vi "SetUpHelper.vi"(8 "ErrorIn":errorcluster, 11 "Reference":T1) -> (0 "ErrorOut":errorcluster, 3 "OutConnection":T1)   [LabVIEW 2019]
uses:
  C:/Users/user/Desktop/lvlib/assemblies/x86/LibraryForLabVIEW.dll
  assemblies/x86/LibraryForLabVIEW.dll
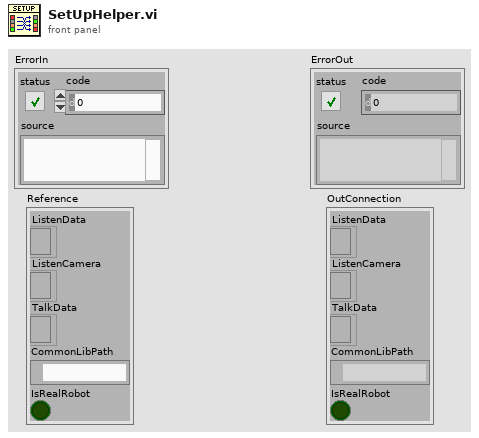
[diagram p1: front panel]
types:
  T1 = cluster{"ListenData":refnum<k24>, "ListenCamera":refnum<k24>, "TalkData":refnum<k24>, "CommonLibPath":path, "IsRealRobot":bool}
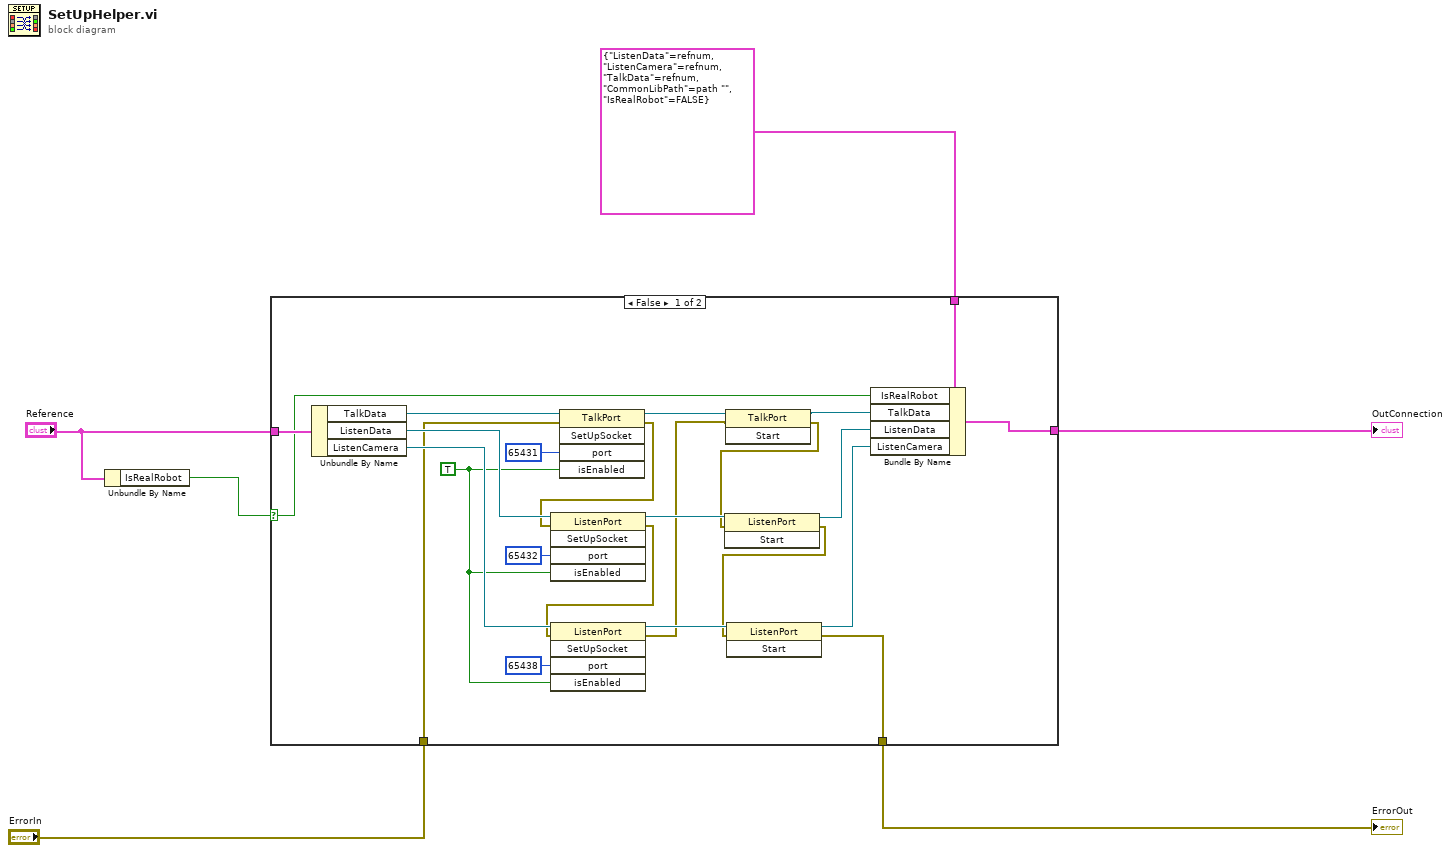
[diagram p0: block diagram]
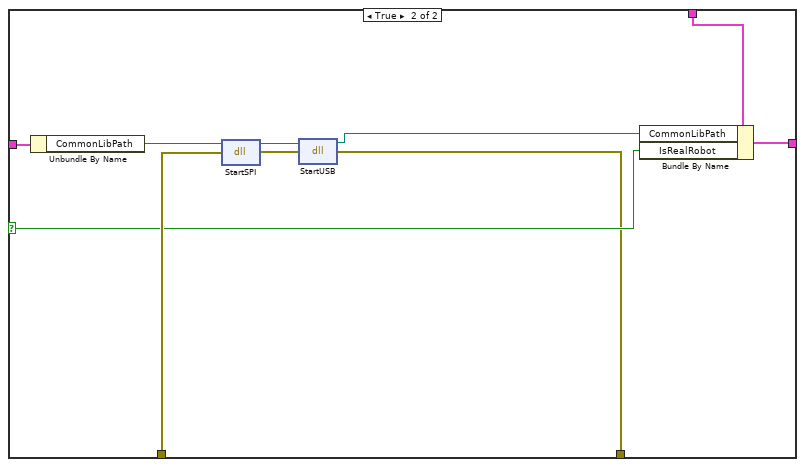
[diagram p2: hidden frame]
diagram:
  n1 = Unbundle By Name("Reference") -> ("IsRealRobot"=w1:bool)
  n2 = case shown="False" w1 {
    selector: w1 -> [w7 w35]
    tunnel: "ErrorIn" -> [w18 w38]
    tunnel: [w11 w31] -> w5
    tunnel: "Reference" -> [w10 w40]
    tunnel: T1 {"ListenData"=refnum, "ListenCamera"=refnum, "TalkData"=refnum, "CommonLibPath"=path "", "IsRealRobot"=FALSE} -> [w9 w37]
    tunnel: [w8 w36] -> w3
    frame False {
      w16 = TRUE
      n3 = Unbundle By Name(w10) -> ("TalkData"=w19:refnum<k24>, "ListenData"=w29:refnum<k24>, "ListenCamera"=w27:refnum<k24>)
      n4 = invoke class="TalkPort" method="SetUpSocket"(reference=w19, error in=w18, "port"=65431, "isEnabled"=w16) -> (reference out=w15:refnum<k24>, error out=w17:errorcluster)  [unwired: 1 in, 3 out]
      n5 = invoke class="ListenPort" method="SetUpSocket"(reference=w29, error in=w17, "port"=65432, "isEnabled"=w16) -> (reference out=w25:refnum<k24>, error out=w26:errorcluster)  [unwired: 1 in, 3 out]
      n6 = invoke class="ListenPort" method="SetUpSocket"(reference=w27, error in=w26, "port"=65438, "isEnabled"=w16) -> (reference out=w24:refnum<k24>, error out=w12:errorcluster)  [unwired: 1 in, 3 out]
      n7 = invoke class="TalkPort" method="Start"(reference=w15, error in=w12) -> (reference out=w14:refnum<k24>, error out=w13:errorcluster)  [unwired: 1 in, 1 out]
      n8 = invoke class="ListenPort" method="Start"(reference=w25, error in=w13) -> (reference out=w22:refnum<k24>, error out=w23:errorcluster)  [unwired: 1 in, 1 out]
      n9 = invoke class="ListenPort" method="Start"(reference=w24, error in=w23) -> (reference out=w21:refnum<k24>, error out=w11:errorcluster)  [unwired: 1 in, 1 out]
      n10 = Bundle By Name(cluster=w9, "IsRealRobot"=w7, "TalkData"=w14, "ListenData"=w22, "ListenCamera"=w21) -> (w8:T1)
    }
    frame True {
      n11 = Unbundle By Name(w40) -> ("CommonLibPath"=w39:path)
      n12 = dll-call lib="?" fn="StartSPI"(path in=w39, error in=w38) -> (path out=w34:path, error out=w33:errorcluster)  [unwired: 2 in]
      n13 = dll-call lib="?" fn="StartUSB"(path in=w34, error in=w33) -> (path out=w32:path, error out=w31:errorcluster)  [unwired: 2 in]
      n14 = Bundle By Name(cluster=w37, "CommonLibPath"=w32, "IsRealRobot"=w35) -> (w36:T1)
    }
  }
  "ErrorOut" <- w5
  "OutConnection" <- w3
